vi "BasePixelCalibSingle.vi"(8 "error in (no error)":errorcluster, 11 "MagSpecCamera in":refnum<class "MagSpecCamera.lvclass">) -> (0 "error out":errorcluster, 3 "MagSpecCamera in":refnum<class "MagSpecCamera.lvclass">)   [LabVIEW 2020, in "MagSpecCamera.lvclass"]
uses:
  MagSpecCamera.lvclass
  OnOffTypeDef.ctl
  MagSpecCamera.lvclass/MagSpecCamera.ctl
  NI_AALPro.lvlib
  NI_AALBase.lvlib
panel:
  out "XY Graph":cluster{"Array out":dbl[], "Array out":dbl[]}(graph)
  out "bending angle Side":dbl[](graph)
  out "bending angle Front":dbl[](graph)
  out "energy dependence":dbl[](graph)
  out "bending angle":dbl[](graph)
  out "pixel angle":dbl[](graph)
  out "position":dbl[](graph)
  out "total path":dbl[](graph)
  out "dp/B":dbl[](graph)
  out "index":dbl[](graph)
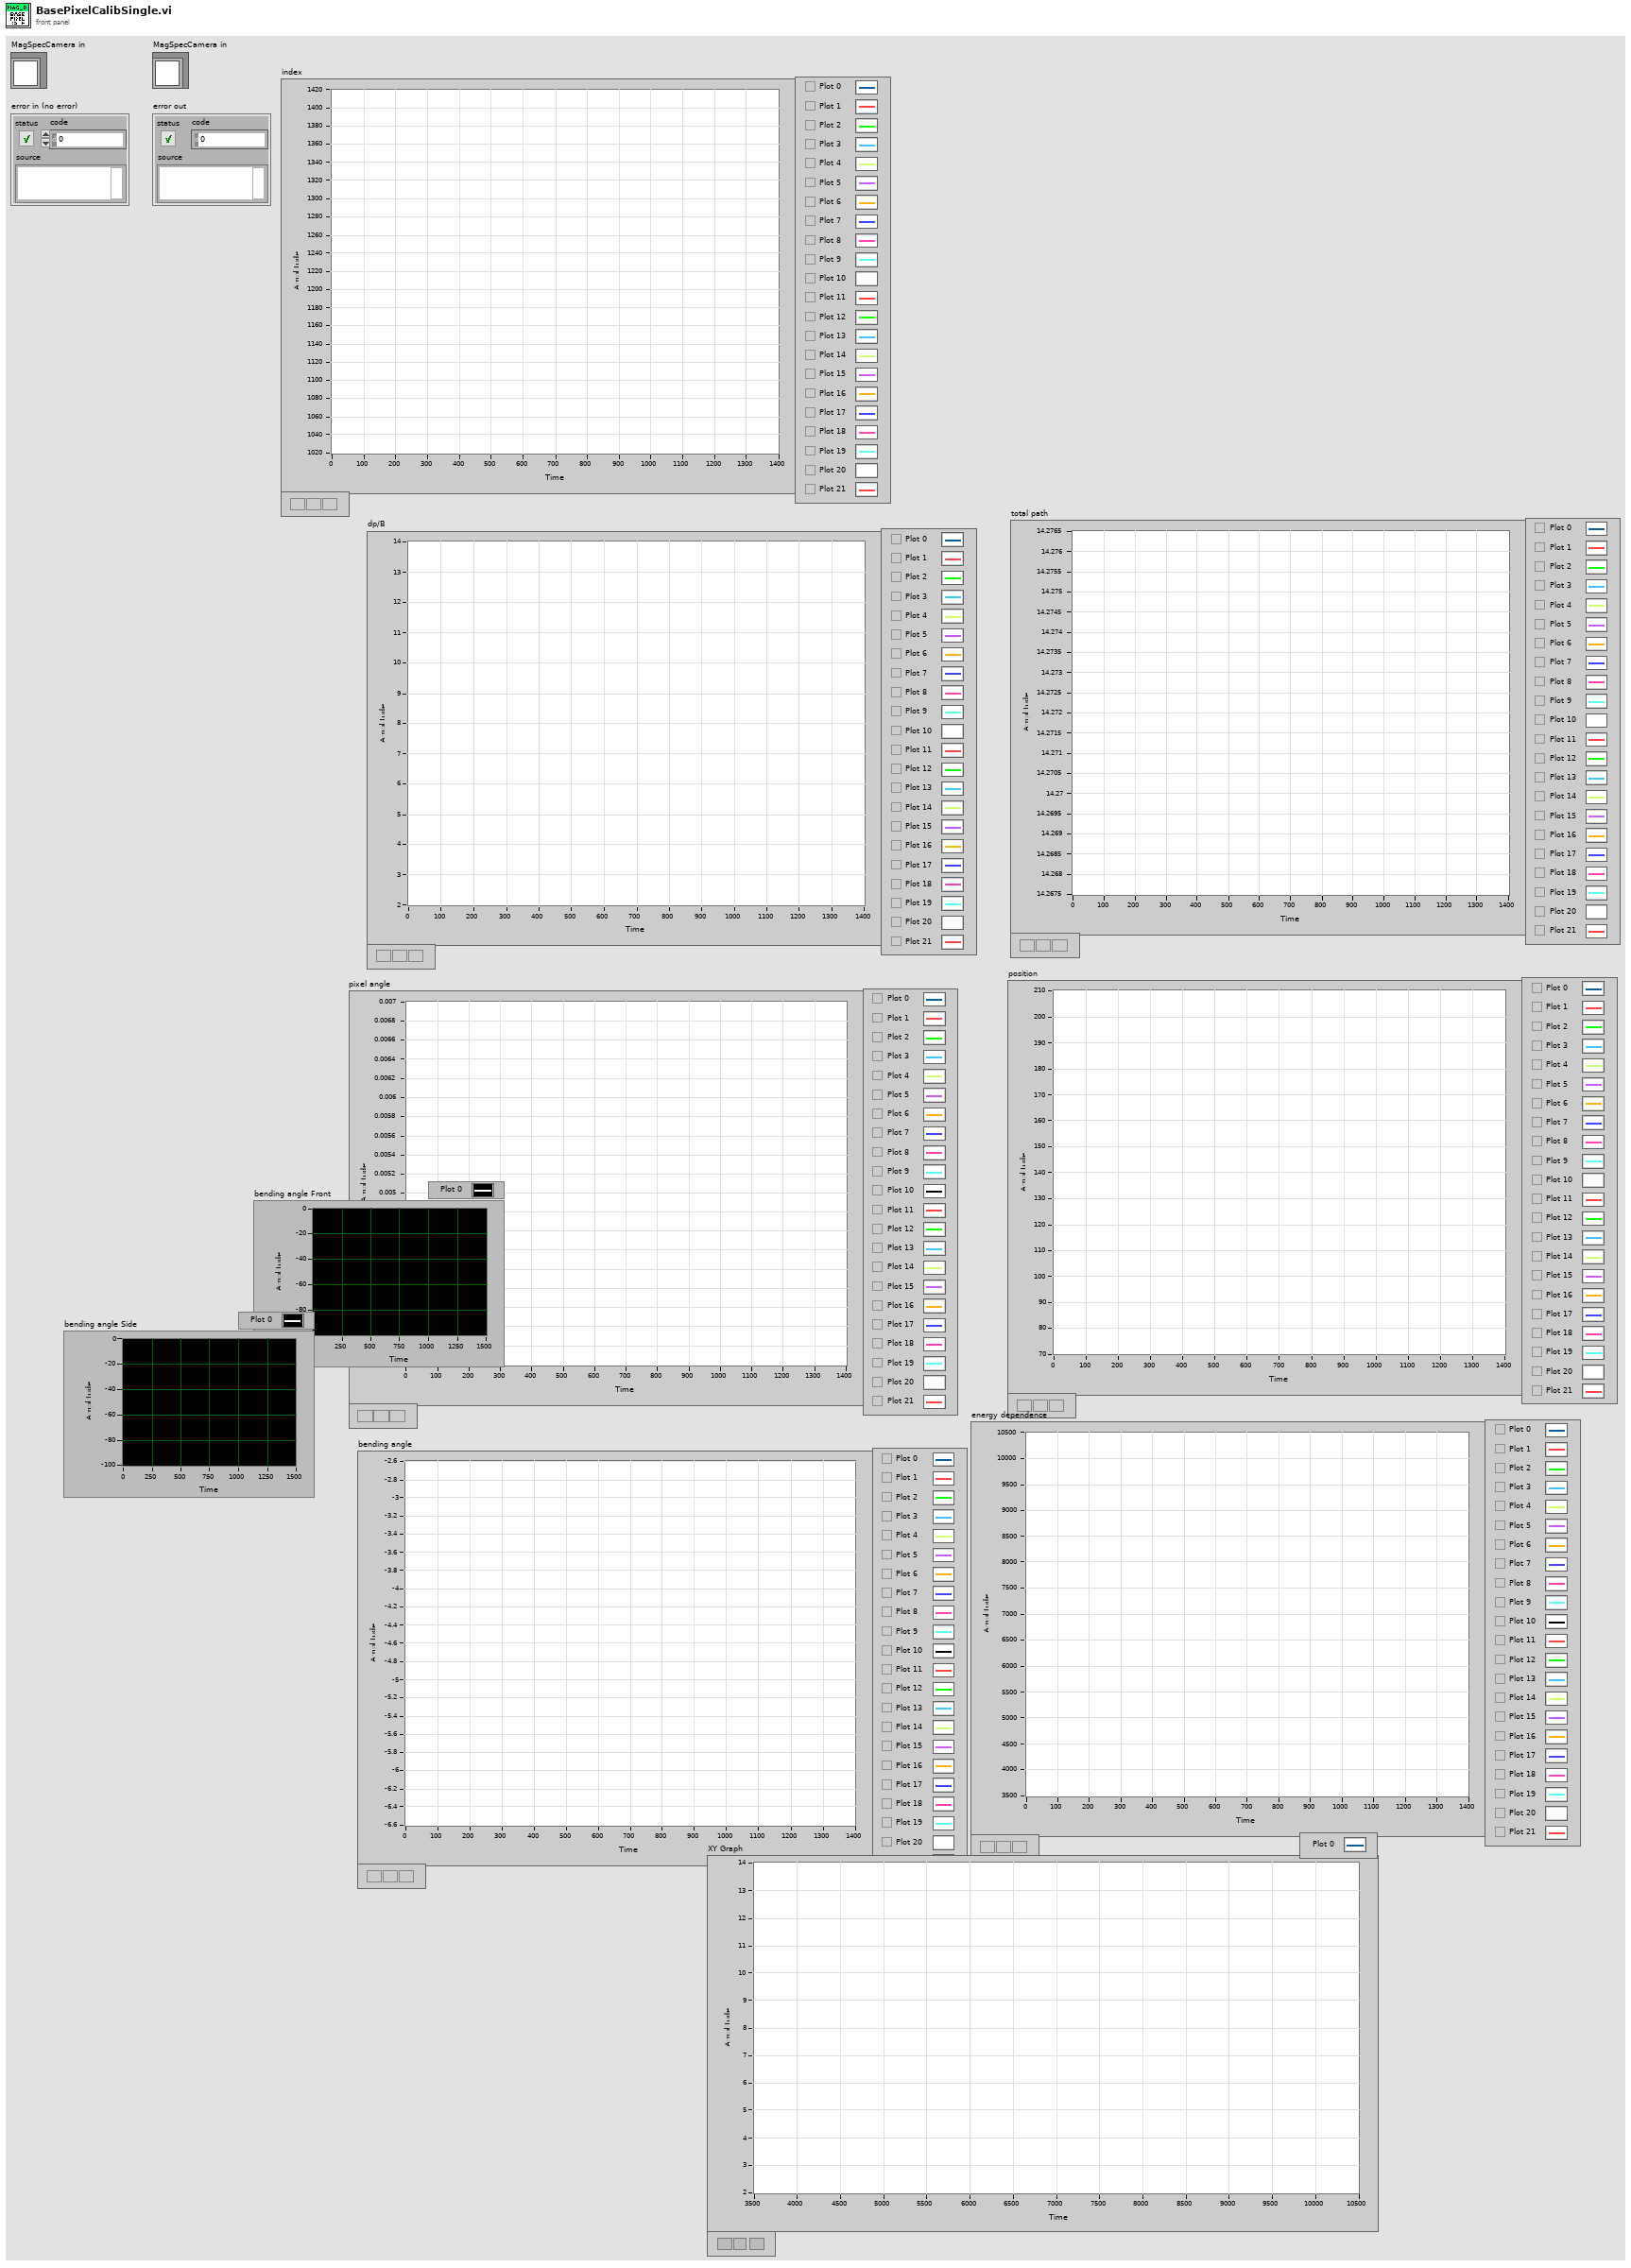
[diagram p1: front panel]
types:
  T1 = typedef "OnOffTypeDef.ctl" = enum16{"off", "on"}
  T2 = typedef "CameraSettings_File.ctl" = cluster{"FOV [mm]":dbl, "Left edge [mm]":dbl, "ROI Y offset":dbl, "ROI height":dbl, "ROI X offset":dbl, "ROI width":dbl, "Y center pixel":dbl, "Y Start":dbl, "Y End":dbl, "X Start":dbl, "X End":dbl, "rot [deg]":dbl}
  T3 = typedef "Calibration_Pixel_based.ctl" = cluster{"y1(pixel)":dbl[], "y2(pixel)":dbl[], "dp/B [MeV/C/B] (pixel)":dbl[], "energyDependence Input(pixel)":dbl[], "bending angle [deg](pixel)":dbl[], "total path(pixel)":dbl[], "pixel angle (y)(pixel)":dbl[], "energy dependence (pixel)":dbl[], "charge compensation (pixel)":dbl[], "Momentum [MeV/C](pixel)":dbl[], "angular compensation(pixel)":dbl[]}
  T4 = typedef "CalibrationCluster.ctl" = cluster{"bending angle Front":dbl[], "bending angle Side":dbl[], "screen [m] Front":dbl[], "screen [m] Side":dbl[], "momentum [MeV/c]":dbl[], "total path [m]":dbl[], "x[mm](rms)":dbl[], "x[mm](rms,b)":dbl[], "y[mm](rms)":dbl[], "y[mm](rms,b)":dbl[]}
  T5 = typedef "OneTimeCalculation.ctl" = cluster{"first Pixel pos [m]":dbl, "Pixel Size [mm]":dbl, "forward":T1}
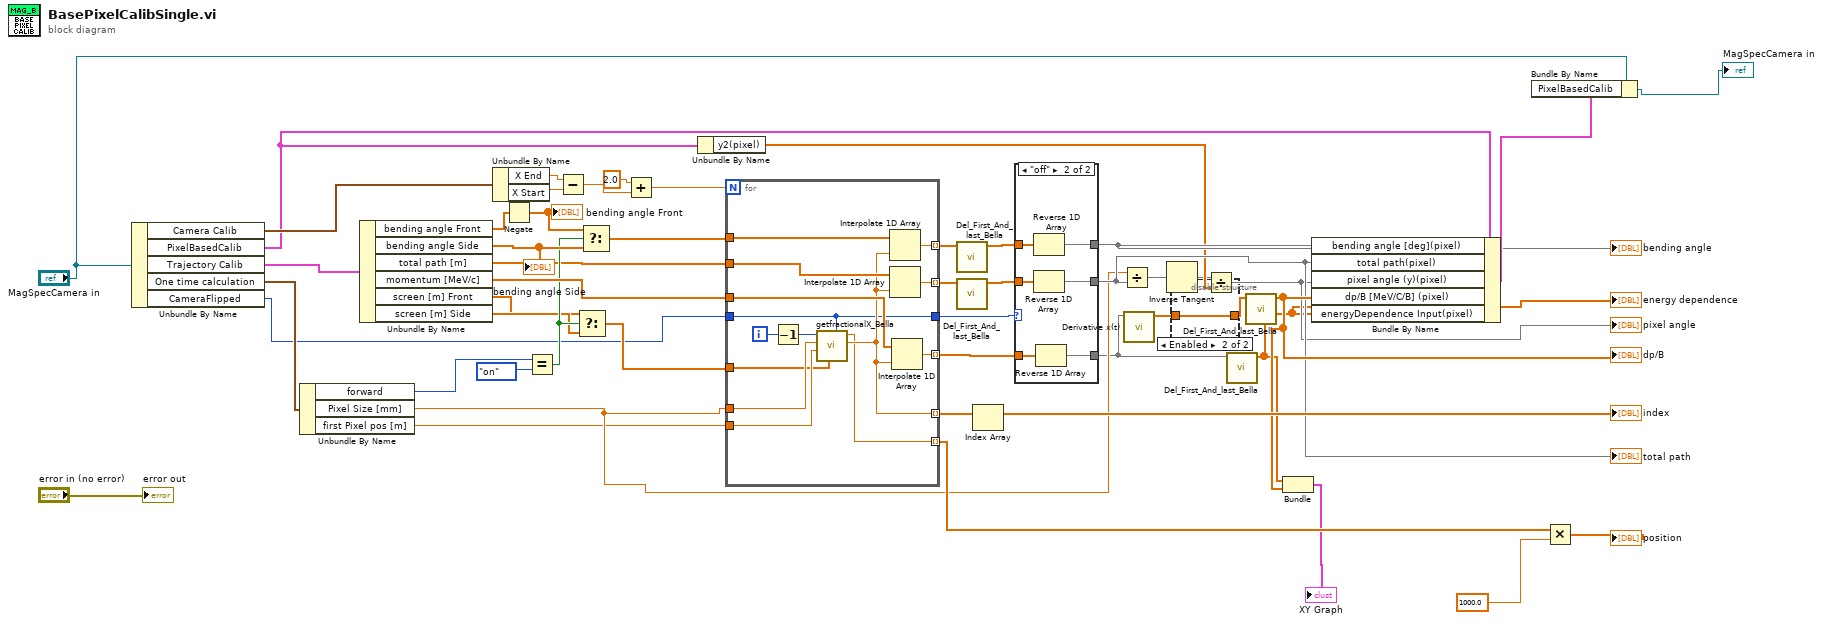
[diagram p0: block diagram]
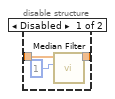
[diagram p2: hidden frame]
diagram:
  n1 = Unbundle By Name("MagSpecCamera in") -> ("Camera Calib"=w43:T2, "PixelBasedCalib"=w3:T3, "Trajectory Calib"=w45:T4, "One time calculation"=w46:T5, "CameraFlipped"=w1:T1)
  n2 = Unbundle By Name(w46) -> ("forward"=w15:T1, "Pixel Size [mm]"=w31:dbl, "first Pixel pos [m]"=w21:dbl)
  n3 = Unbundle By Name(w45) -> ("bending angle Front"=w5:dbl[], "bending angle Side"=w20:dbl[], "total path [m]"=w7:dbl[], "momentum [MeV/c]"=w16:dbl[], "screen [m] Front"=w10:dbl[], "screen [m] Side"=w11:dbl[])
  "bending angle Side" <- w20
  n4 = Unbundle By Name(w43) -> ("X End"=w9:dbl, "X Start"=w8:dbl)
  n5 = Negate(x=w5) -> (-x=w4:dbl[])
  "bending angle Front" <- w4
  n6 = Equal?(x=w15, y=OnOffTypeDef."on") -> (x = y?=w14:bool)
  n7 = Subtract(x=w9, y=w8) -> (x-y=w42:dbl)
  n8 = Select(t=w10, s=w14, f=w11) -> (s? t:f=w13:dbl[])
  n9 = Select(t=w4, s=w14, f=w20) -> (s? t:f=w19:dbl[])
  n10 = Add(x=2.0, y=w42) -> (x+y=w12:dbl)
  n11 = Unbundle By Name(w3) -> ("y2(pixel)"=w32:dbl[])
  n12 = for {
    N: w12 -> [_]
    tunnel: w31 -> [w64]
    tunnel: w21 -> [w63]
    tunnel: w19 -> [w62]
    tunnel: [w61] -> w24 mode=indexing
    tunnel: w16 -> [w60]
    tunnel: [w59] -> w2 mode=indexing
    tunnel: w7 -> [w55]
    tunnel: [w58] -> w29 mode=indexing
    tunnel: w1 -> [w52]
    tunnel: [w52] -> w6
    tunnel: [w54] -> w44 mode=indexing
    tunnel: w13 -> [w53]
    tunnel: [w51] -> w39 mode=indexing
    i -> [w57]
    n13 = Decrement(x=w57) -> (x-1=w56:i32)
    n14 = call "getfractionalX_Bella.vi"("CameraFlipped"=w52, "screen [m]"=w53, "position [m]"=w63, "pixelsize"=w64, "position index"=w56) -> ("index"=w54:dbl, "position m"=w51:dbl)  [unwired: 5 in]
    n15 = Interpolate 1D Array(1:w54, 2:w62) -> (0:w61:dbl)
    n16 = Interpolate 1D Array(1:w54, 2:w55) -> (0:w58:dbl)
    n17 = Interpolate 1D Array(1:w54, 2:w60) -> (0:w59:dbl)
  }
  "index" <- w44
  n18 = call "Del_First_And_last_Bella.vi"("Array in"=w24) -> ("Array out"=w25:dbl[])  [unwired: 10 in]
  n19 = call "Del_First_And_last_Bella.vi"("Array in"=w29) -> ("Array out"=w30:dbl[])  [unwired: 10 in]
  n20 = Index Array(array=w44) -> ()  [unwired: 1 in, 1 out]
  n21 = case shown="\"off\"" w6 {
    tunnel: w30 -> [w66 w73]
    tunnel: [w67 w72] -> w35
    tunnel: [w66 w71] -> w40
    tunnel: w25 -> [w67 w70]
    tunnel: [w65 w69] -> w17
    tunnel: w2 -> [w65 w68]
    frame "on" {
    }
    frame "off" {
      n22 = Reverse 1D Array(array=w70) -> (reversed array=w72:dbl[])
      n23 = Reverse 1D Array(array=w73) -> (reversed array=w71:dbl[])
      n24 = Reverse 1D Array(array=w68) -> (reversed array=w69:dbl[])
    }
  }
  "total path" <- w40
  "bending angle" <- w35
  n25 = Divide(x=w31, y=w40) -> (x/y=w22:dbl[])
  n26 = call "Derivative x(t).vi"("X"=w17) -> ("dX/dt"=w27:dbl[])  [unwired: 9 in, 1 out]
  n27 = Inverse Tangent(1:w22) -> (0:w23:dbl[])
  n28 = disable-structure shown="Enabled" {
    disable-tunnel: [w76 w77] -> w28
    disable-tunnel: w27 -> [w75 w77]
    frame Disabled {
      n29 = call "Median Filter.vi"("left rank"=1, "X"=w75) -> ("Filtered X"=w76:dbl[])  [unwired: 8 in, 1 out]
    }
    frame Enabled {
    }
  }
  n30 = Divide(x=w23, y=w32) -> (x/y=w36:dbl[])
  "pixel angle" <- w36
  n31 = call "Del_First_And_last_Bella.vi"("Array in"=w17) -> ("Array out"=w34:dbl[])  [unwired: 10 in]
  "energy dependence" <- w34
  n32 = call "Del_First_And_last_Bella.vi"("Array in"=w28) -> ("Array out"=w41:dbl[])  [unwired: 10 in]
  "dp/B" <- w41
  n33 = Bundle("Array out"=w34, "Array out"=w41) -> (→"XY Graph":cluster{"Array out":dbl[], "Array out":dbl[]})  [unwired: 1 in]
  n34 = Bundle By Name(cluster=w3, "bending angle [deg](pixel)"=w35, "total path(pixel)"=w40, "pixel angle (y)(pixel)"=w36, "dp/B [MeV/C/B] (pixel)"=w41, "energyDependence Input(pixel)"=w34) -> (w47:T3)
  n35 = Bundle By Name(cluster="MagSpecCamera in", "PixelBasedCalib"=w47) -> (→"MagSpecCamera in":refnum<class "MagSpecCamera.lvclass">)
  n36 = Multiply(x=w39, y=1000.0) -> (x*y=→"position":dbl[])
  "error out" <- "error in (no error)"
